vi "HRTF-Read HRTF Matfile.vi"(0 "path":path, 11 "Error In":errorcluster) -> (8 "filt":T1, 15 "error out":errorcluster)   [LabVIEW 2020]
uses:
  Typedefs/HRTF-filt Cluster.ctl
  <userlib>/_matio/level5/Public/Read/Extract Data Element.llb/Extract Data Element (Anything).vi
  <userlib>/_matio/level5.lvlib
panel:
  out "b":dbl[](array[numeric])
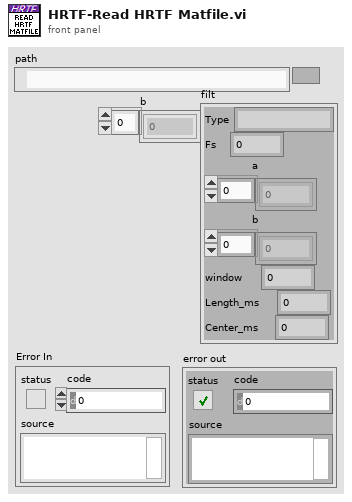
[diagram p1: front panel]
types:
  T1 = typedef "HRTF-filt Cluster.ctl" = cluster{"Type":string, "Fs":dbl, "a":dbl[], "b":dbl[], "window":i32, "Length_ms":dbl, "Center_ms":dbl}
  T2 = cluster{"Type":string, "Fs":dbl, "a":dbl[], "b":dbl[]}
  T3 = enum16{"big-endian, network order", "native, host order", "little-endian"}
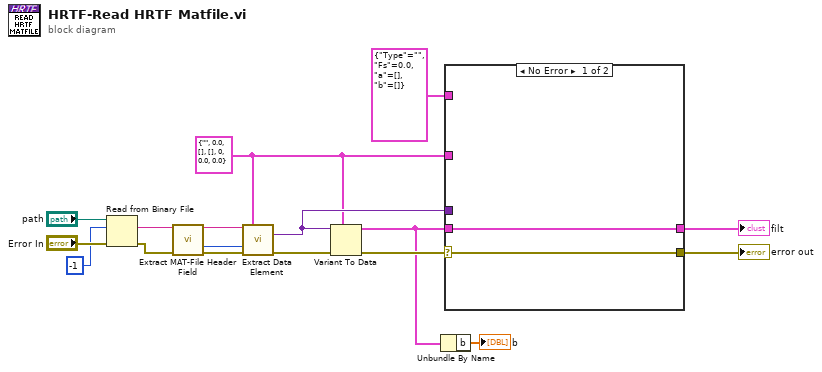
[diagram p0: block diagram]
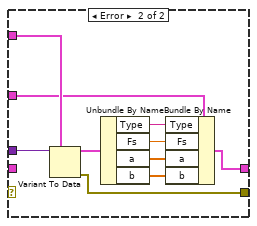
[diagram p2: hidden frame]
diagram:
  w3 = T1 {"Type"="", "Fs"=0.0, "a"=[], "b"=[], "window"=0, "Length_ms"=0.0, "Center_ms"=0.0} ("data")
  n1 = Read from Binary File(8:"Error In", 10:-1 ("count (1)"), 11:"path") -> (0:w13:errorcluster, 2:w10:string)  [unwired: 3 in, 2 out]
  n2 = call <userlib>:"Extract MAT-File Header Field.vi"("string"=w10, "error in (no error)"=w13) -> ("resulting string"=w16:string, "endian indicator"=w17:T3, "error out"=w14:errorcluster)  [unwired: 8 in, 3 out]
  n3 = call-poly <userlib>:"Extract Data Element.vi"("string"=w16, "type"=w3, "byte order (0:big-endian, network order)"=w17, "error in"=w14) -> ("data"=w5:variant, "error out"=w15:errorcluster)  [unwired: 8 in, 2 out]
  n4 = Variant To Data(error in=w15, type=w3, Variant=w5) -> (data=w2:T1, error out=w8:errorcluster)
  n5 = Unbundle By Name(w2) -> ("b"=→"b":dbl[])
  n6 = case shown="No Error" w8 {
    selector: w8 -> [w18 _]
    tunnel: w2 -> [w19 _]
    tunnel: [w19 w21] -> w7
    tunnel: [w18 w20] -> w6
    tunnel: w5 -> [_ w29]
    tunnel: T2 {"Type"="", "Fs"=0.0, "a"=[], "b"=[]} ("data") -> [_ w28]
    tunnel: w3 -> [_ w26]
    frame No Error {
    }
    frame Error {
      n7 = Variant To Data(type=w28, Variant=w29) -> (data=w27:T2, error out=w20:errorcluster)  [unwired: 1 in]
      n8 = Unbundle By Name(w27) -> ("Type"=w25:string, "Fs"=w24:dbl, "a"=w23:dbl[], "b"=w22:dbl[])
      n9 = Bundle By Name(cluster=w26, "Type"=w25, "Fs"=w24, "a"=w23, "b"=w22) -> (w21:T1)
    }
  }
  "error out" <- w6
  "filt" <- w7
